vi "Check Params Changed.vi"(7 "UI Ref":refnum<vi>, 10 "Alias":string, 11 "Settings in":T1) -> (2 "New Flatterned Params (Empty if no change)":string, 3 "Settings out":T1={"Step Values"=[], "Only Execute When Test Running"=TRUE, "Reset Sequence When Test Starts"=TRUE, "Current Sequence ID"=0, "Total Iterations"=0, "Current Step Start Timestamp"=0.0, "Number of Sequence Steps"=0, "Num of Analog Channels"=0, "Num of Digital Channels"=0, "Delay Before Starting Sequence"=0.0, "Show UI"=FALSE, "Time Remaining"=0.0, "Test Running"=FALSE, "Pause Timestamp"=0.0})   [LabVIEW 2020, in "Sequencer with Output Values.lvlib" / "Sequencer with Output Values.lvclass"]
uses:
  Sequencer with Output Values.lvclass
  Params.ctl
  Step Settings.ctl
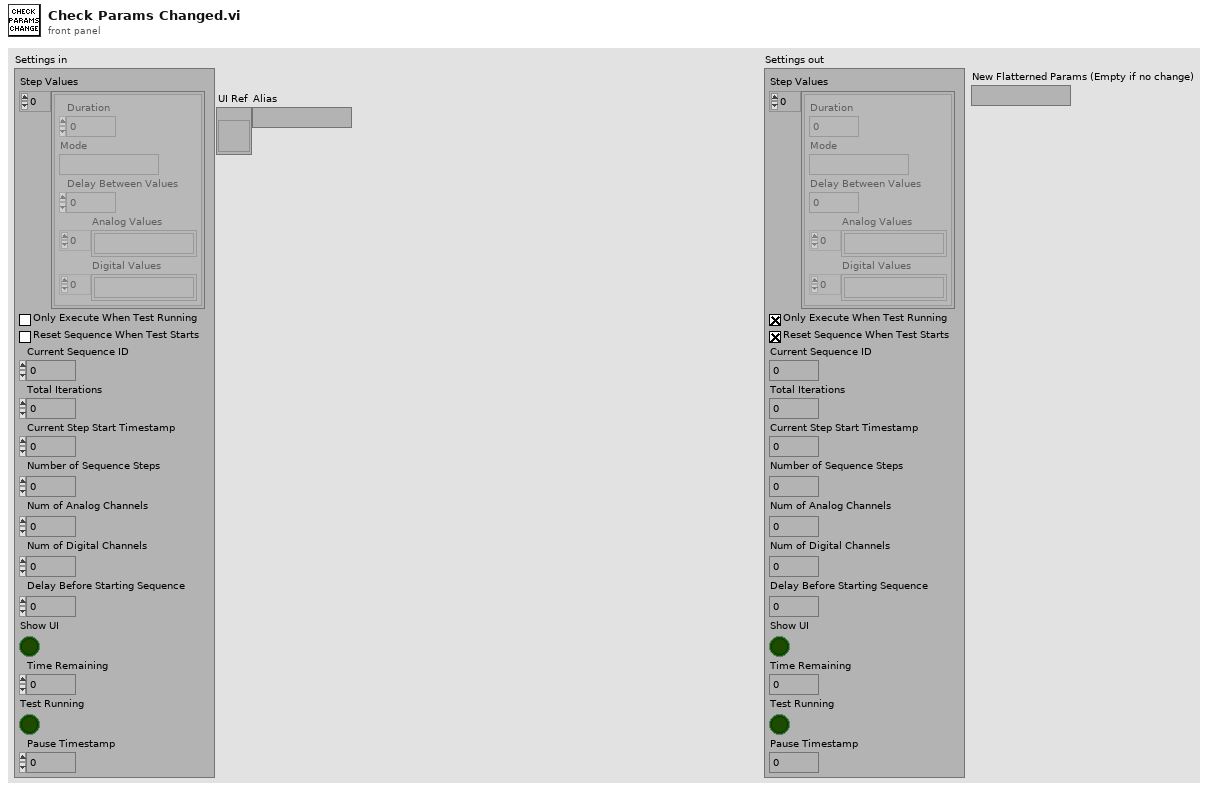
[diagram p1: front panel]
types:
  T1 = typedef "Sequencer with Output Values.lvlib/Sequencer with Output Values.lvclass/Params.ctl" = cluster{"Step Values":T2[], "Only Execute When Test Running":bool, "Reset Sequence When Test Starts":bool, "Current Sequence ID":u32, "Total Iterations":u32, "Current Step Start Timestamp":dbl, "Number of Sequence Steps":i32, "Num of Analog Channels":i32, "Num of Digital Channels":i32, "Delay Before Starting Sequence":dbl, "Show UI":bool, "Time Remaining":dbl, "Test Running":bool, "Pause Timestamp":dbl}
  T2 = typedef "Sequencer with Output Values.lvlib/Sequencer with Output Values.lvclass/Step Settings.ctl" = cluster{"Duration":dbl, "Mode":string, "Delay Between Values":dbl, "Analog Values":string[], "Digital Values":string[]}
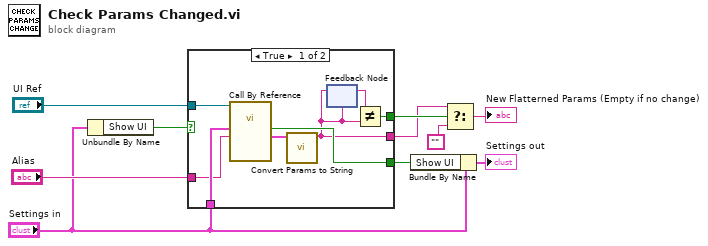
[diagram p0: block diagram]
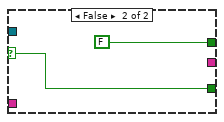
[diagram p2: hidden frame]
diagram:
  n1 = Unbundle By Name("Settings in") -> ("Show UI"=w8:bool)
  n2 = case shown="True" w8 {
    selector: w8 -> [_ w19]
    tunnel: "UI Ref" -> [w18 _]
    tunnel: "Settings in" -> [w17 _]
    tunnel: "Alias" -> [w16 _]
    tunnel: [w13 FALSE] -> w4
    tunnel: [w15 w19] -> w6
    tunnel: [w11 _] -> w3
    frame True {
      n3 = call-by-ref "?"(reference=w18, "Alias"=w16, "Init Settings In"=w17) -> ("Applied Settings"=w14:T1, "Show UI"=w15:bool)  [unwired: 9 in, 2 out]
      n4 = call "Convert Params to String.vi"("Settings"=w14) -> ("String out"=w11:string)  [unwired: 10 in]
      n5 = feedback #1(w11) -> (w12:string)
      n6 = feedback-in #1(w11) -> ()
      n7 = Not Equal?(x=w12, y=w11) -> (x != y?=w13:bool)
    }
    frame False {
    }
  }
  n8 = Bundle By Name(cluster="Settings in", "Show UI"=w6) -> (→"Settings out":T1)
  n9 = Select(t=w3, s=w4, f="") -> (s? t:f=→"New Flatterned Params (Empty if no change)":string)
